vi "calibrateWaveplatePhotons.vi"() -> ()   [LabVIEW 2013]
uses:
  <vilib>/Utility/file.llb/Write To Spreadsheet File (DBL).vi
panel:
  in  "GPIB address":string="15"
  in  "Report":enum16{"Time to reach count", "Trigger rate"}(ring)
  in  "Start position":dbl
  out "Data":dbl[][](array[numeric])
  in  "Write to file?":bool
  out "error out":errorcluster
  in  "Photon number":dbl
  in  "Repetitions":dbl=1.0
  in  "file path (dialog if empty)":path
  out "XY Graph":cluster{"Y":dbl[], "Y":dbl[]}[](graph)
  in  "Stop position":dbl=180.0
  in  "Rotation increment":dbl=10.0 format="%.2f"
  out "Current position (units)":dbl format="%.2f"
  in  "Axis in":i32=3
  in  "Timeout (ms)":u32=500
  in  "SerialPort":u8=3
  in  "stop":bool
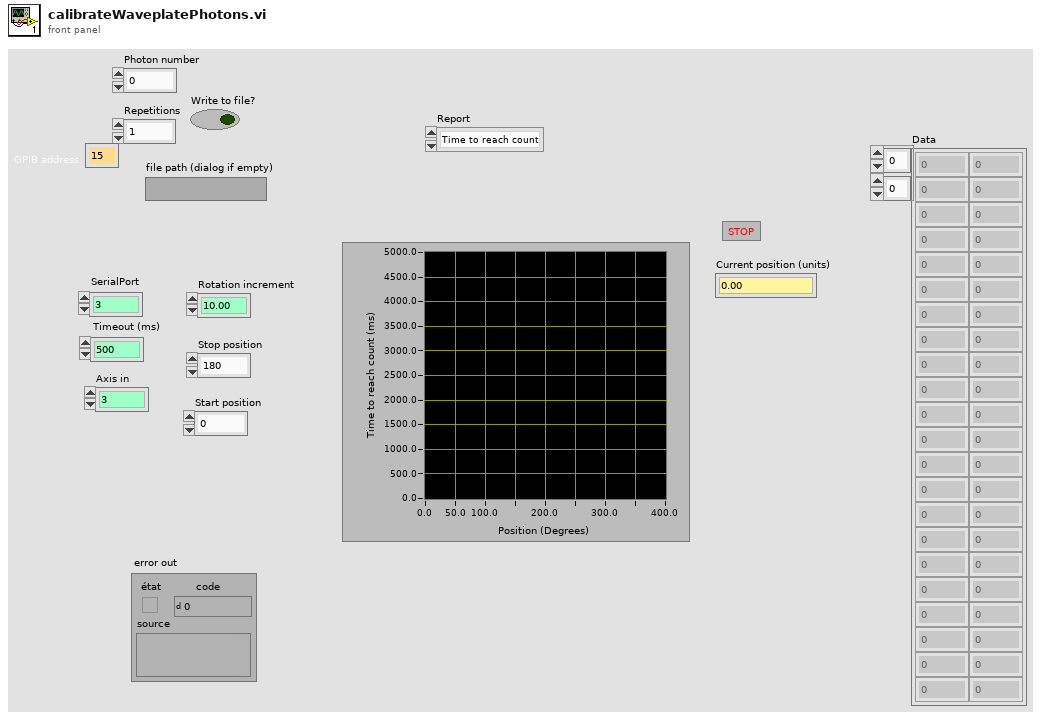
[diagram p1: front panel]
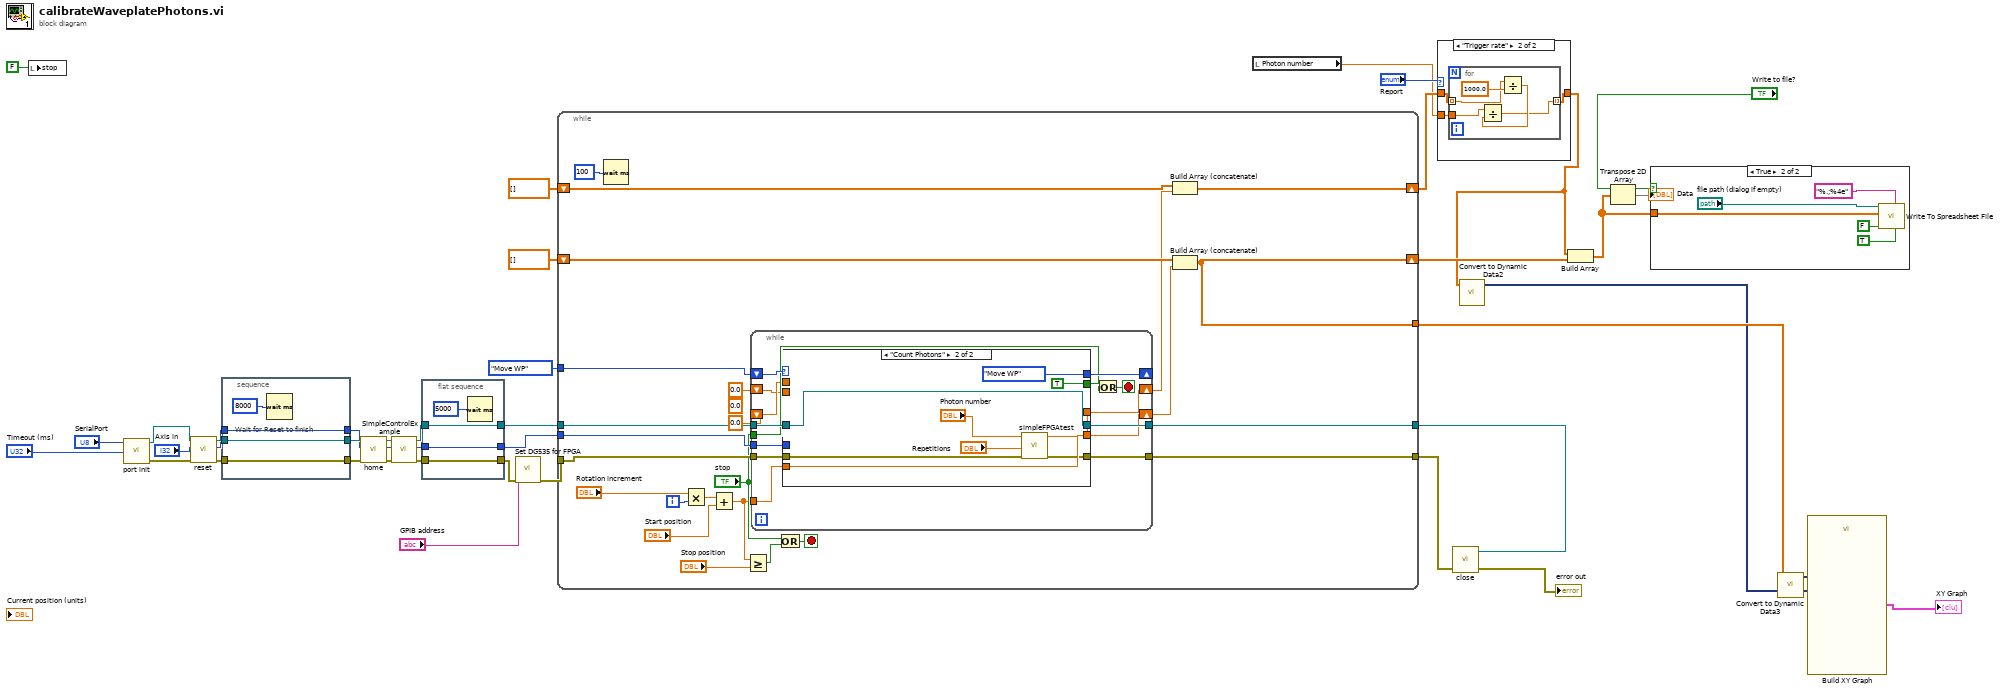
[diagram p0: block diagram]
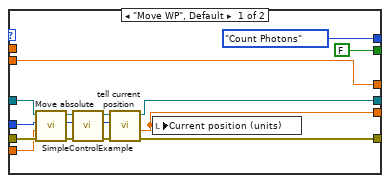
[diagram p4: hidden frame]
diagram:
  n1 = local write "stop"(FALSE ("stop")) -> ()
  n2 = call "port init.vi"("Timeout (ms)"="Timeout (ms)", "SerialPort"="SerialPort") -> ("error out"=w35:errorcluster, "Visa Handle"=w34:refnum<visa-resource-name>)  [unwired: 2 in]
  n3 = call "reset.vi"("error in"=w35, "Axis in"="Axis in", "VISA Handle in"=w34) -> ("error out"=w32:errorcluster, "Axis out"=w27:i32, "VISA Handle out"=w29:refnum<visa-resource-name>)  [unwired: 3 in, 1 out]
  n4 = stacked-sequence {
    tunnel: w32 -> [w44]
    tunnel: [w44] -> w31
    tunnel: [w43] -> w28
    tunnel: w29 -> [w43]
    tunnel: w27 -> [w42]
    tunnel: [w42] -> w26
    frame #0 {
      # "Wait for Reset to finish"
      n5 = Wait (ms)(milliseconds to wait=u32 8000) -> ()  [unwired: 1 out]
    }
  }
  n6 = call "home.vi"("error in"=w31, "Axis in"=w26, "VISA Handle in"=w28) -> ("error out"=w37:errorcluster, "Axis out"=w36:i32, "VISA Handle out"=w38:refnum<visa-resource-name>)  [unwired: 3 in, 1 out]
  n7 = call "SimpleControlExample.vi"("error in"=w37, "Axis in"=w36, "VISA Handle in"=w38) -> ("error out"=w21:errorcluster, "Axis out"=w25:i32, "VISA Handle out"=w23:refnum<visa-resource-name>)  [unwired: 2 in, 2 out]
  n8 = flat-sequence {
    tunnel: w25 -> [w49]
    tunnel: [w49] -> w24
    tunnel: w23 -> [w48]
    tunnel: [w48] -> w22
    tunnel: w21 -> [w47]
    tunnel: [w47] -> w3
    frame #0 {
      n9 = Wait (ms)(milliseconds to wait=u32 5000) -> ()  [unwired: 1 out]
    }
  }
  n10 = call "Set DG535 for FPGA.vi"("error in (no error)"=w3, "GPIB address"="GPIB address") -> ("error out"=w2:errorcluster)  [unwired: 9 in]
  n11 = while {
    tunnel: enum16{"Move WP", "Count Photons", "Stop"}."Move WP" -> [w73]
    tunnel: w22 -> [w72]
    tunnel: w24 -> [w71]
    tunnel: w2 -> [w70]
    tunnel: [w64] -> w30
    tunnel: [w63] -> w19
    shift-right: [w51] -> w6
    shift-left: dbl[] [] -> [w60]
    shift-right: [w50] -> w16
    shift-left: dbl[] [] -> [w58]
    tunnel: [w50] -> w11
    i -> [w62]
    stop <- w65 stop-if-true
    (unwired) 0.0 ("Photon number")
    n12 = Wait (ms)(milliseconds to wait=u32 100) -> ()  [unwired: 1 out]
    n13 = Multiply(x="Rotation increment", y=w62) -> (x*y=w56:dbl)
    n14 = Add(x=w56, y="Start position") -> (x+y=w54:dbl)
    n15 = Greater Or Equal?(x=w54, y="Stop position") -> (x >= y?=w67:bool)
    n16 = while {
      shift-right: [w87] -> _
      shift-left: w73 -> [w88]
      tunnel: w72 -> [w86]
      tunnel: w71 -> [w85]
      tunnel: w70 -> [w84]
      tunnel: [w83] -> w63
      tunnel: [w82] -> w64
      tunnel: w54 -> [w79]
      tunnel: "stop" -> [w78]
      shift-right: [w77] -> w59
      shift-left: 0.0 ("Current position (units)") -> [w76]
      shift-right: [w75] -> w57
      shift-left: 0.0 ("Value") -> [w74]
      stop <- w80 stop-if-true
      n17 = case shown="\"Count Photons\"" w88 {
        tunnel: [enum16{"Move WP", "Count Photons", "Stop"}."Count Photons" enum16{"Move WP", "Count Photons", "Stop"}."Move WP"] -> w87
        tunnel: w86 -> [w98 w111]
        tunnel: w85 -> [w97 _]
        tunnel: w84 -> [w96 w107]
        tunnel: [w95 w106] -> w83
        tunnel: [w94 w111] -> w82
        tunnel: [FALSE ("x") TRUE ("x")] -> w81
        tunnel: w79 -> [w92 w110]
        tunnel: [w91 w110] -> w77
        tunnel: w76 -> [_ _]
        tunnel: [w89 w105] -> w75
        tunnel: w74 -> [w89 _]
        frame "Move WP", Default {
          n18 = call "Move absolute.vi"("error in"=w96, "New target position (units)"=w92, "Axis in"=w97, "VISA Handle in"=w98) -> ("error out"=w99:errorcluster, "Axis out"=w100:i32, "VISA Handle out"=w101:refnum<visa-resource-name>)  [unwired: 2 in, 1 out]
          n19 = call "SimpleControlExample.vi"("error in"=w99, "Axis in"=w100, "VISA Handle in"=w101) -> ("error out"=w102:errorcluster, "Axis out"=w103:i32, "VISA Handle out"=w104:refnum<visa-resource-name>)  [unwired: 2 in, 2 out]
          n20 = call "tell current position.vi"("error in"=w102, "Axis in"=w103, "VISA Handle in"=w104) -> ("error out"=w95:errorcluster, "Current position (units)"=w91:dbl, "VISA Handle out"=w94:refnum<visa-resource-name>)  [unwired: 2 in, 2 out]
          n21 = local write "Current position (units)"(w91) -> ()
        }
        frame "Count Photons" {
          n22 = call "simpleFPGAtest.vi"("error in"=w107, "Repetitions"="Repetitions", "Photon number"="Photon number") -> ("error IO"=w106:errorcluster, "Time"=w105:dbl)  [unwired: 3 in]
        }
      }
      n23 = Or(x=w81, y=w78) -> (x .or. y?=w80:bool)
    }
    n24 = Or(x="stop", y=w67) -> (x .or. y?=w65:bool)
    n25 = Build Array (concatenate)(w60, w57) -> (w51:dbl[])
    n26 = Build Array (concatenate)(w58, w59) -> (w50:dbl[])
  }
  n27 = local read "Photon number"() -> (w4:dbl)
  n28 = case shown="\"Trigger rate\"" "Report" {
    tunnel: w6 -> [w114 w117]
    tunnel: [w114 w116] -> w5
    tunnel: w4 -> [_ w115]
    frame "Time to reach count", Default {
    }
    frame "Trigger rate" {
      n29 = for {
        tunnel: w117 -> [w121] mode=indexing
        tunnel: [w119] -> w116 mode=indexing
        tunnel: w115 -> [w118]
        n30 = Divide(x=w121, y=1000.0) -> (x/y=w120:dbl)
        n31 = Divide(x=w118, y=w120) -> (x/y=w119:dbl)
      }
    }
  }
  n32 = call "close.vi"("error in"=w19, "VISA Handle in"=w30) -> ("error out"=→"error out":errorcluster)  [unwired: 3 in]
  n33 = call "Convert to Dynamic Data2"("Array"=w5) -> ("Dynamic Data Type"=w9:dynamicdata)  [unwired: 3 in]
  n34 = Build Array(w5, w16) -> (w14:dbl[][])
  n35 = Transpose 2D Array(2D array=w14) -> (transposed array=→"Data":dbl[][])
  n36 = case shown="True" "Write to file?" {
    tunnel: w14 -> [_ w123]
    frame False {
    }
    frame True {
      n37 = call-poly <vilib>:"Write To Spreadsheet File.vi"("transpose? (no:F)"=TRUE, "format (%.3f)"="%.;%4e", "append to file? (new file:F)"=FALSE, "2D data"=w123, "file path (dialog if empty)"="file path (dialog if empty)") -> ()  [unwired: 3 in, 1 out]
    }
  }
  n38 = call "Convert to Dynamic Data3"("Array"=w11) -> ("Dynamic Data Type"=w7:dynamicdata)  [unwired: 3 in]
  n39 = call "Build XY Graph"("Y Input"=w9, "X Input"=w7) -> ("XY Graph"=→"XY Graph":cluster{"Y":dbl[], "Y":dbl[]}[])  [unwired: 3 in, 6 out]
